vi "PulseProp.vi"(0 "Data":dbl[](array[numeric]) format="%.2f", 1 "Scale factor":dbl format="%.2f", 2 "spacing":dbl format="%.2f") -> (6 "Pts in range":dbl format="%.2f", 7 "width":dbl format="%.2f", 8 "StopValue":dbl format="%.2f", 9 "Start pt":i32, 10 "StartValue":dbl format="%.2f")   [LabVIEW 2022 SP3]
panel:
  out "Waveform Graph":dbl[](graph)
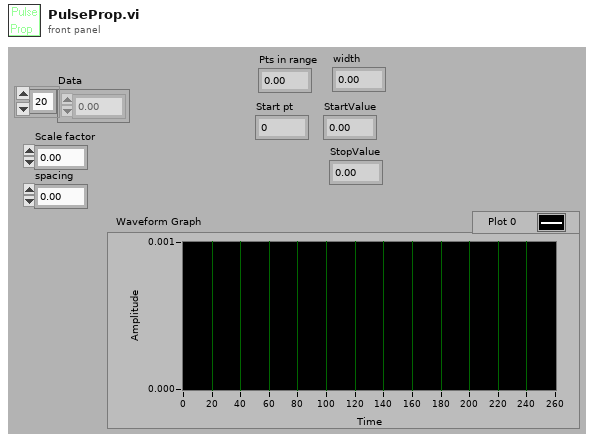
[diagram p1: front panel]
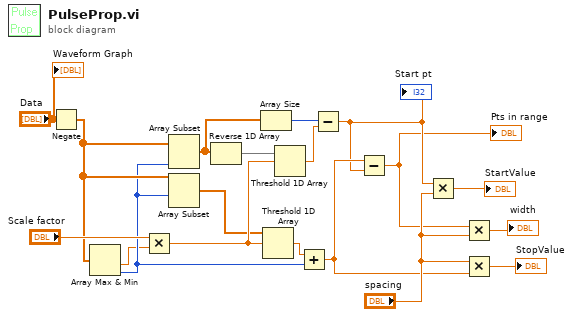
[diagram p0: block diagram]
diagram:
  n1 = Negate(x="Data") -> (-x=w5:dbl[])
  n2 = Array Max & Min(array=w5) -> (min value=w3:dbl, min index (indices)=w4:i32)  [unwired: 2 out]
  n3 = Multiply(x="Scale factor", y=w3) -> (x*y=w18:dbl)
  n4 = Array Subset(array=w5, length=w4) -> (w2:dbl[])  [unwired: 1 in]
  n5 = Array Subset(array=w5, index=w4) -> (w6:dbl[])  [unwired: 1 in]
  n6 = Reverse 1D Array(array=w2) -> (reversed array=w7:dbl[])
  n7 = Array Size(array=w2) -> (size(s)=w16:i32)
  n8 = Threshold 1D Array(2:w18, 3:w6) -> (0:w17:dbl)  [unwired: 1 out]
  n9 = Threshold 1D Array(2:w18, 3:w7) -> (0:w15:dbl)  [unwired: 1 out]
  n10 = Add(x=w17, y=w4) -> (x+y=w12:dbl)
  n11 = Subtract(x=w16, y=w15) -> (x-y=w11:dbl)
  "Start pt" <- w11
  n12 = Subtract(x=w12, y=w11) -> (x-y=w10:dbl)
  "Pts in range" <- w10
  n13 = Multiply(x=w11, y="spacing") -> (x*y=→"StartValue":dbl)
  n14 = Multiply(x=w10, y="spacing") -> (x*y=→"width":dbl)
  n15 = Multiply(x="spacing", y=w12) -> (x*y=→"StopValue":dbl)
  "Waveform Graph" <- "Data"
